vi "64x48_Frame1.vi"   [LabVIEW 2014]
uses:
  QwaveSys_Interface/QwaveSys_Interface.lvlib
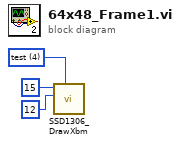
[diagram p0: block diagram]
diagram:
  w1 = u16 4 items=["WiFi Logo", "Active Symbole", "Inactive Symbole", "NETPIE", "test"] ("xbm")
  n1 = call "SSD1306_DrawXbm.vi"("xbm"=w1, "y"=u8 12, "x"=u8 15) -> ()  [unwired: 8 in, 1 out]
